vi "Read Config.vi"(8 "error in (no error)":errorcluster, 11 "Path":path) -> (0 "error out":errorcluster, 2 "Config":T1, 3 "File Created?":bool)   [LabVIEW 2020, in "MacroAssert.lvlib"]
doc: "Reads a config file located at <B>Path</B>."
uses:
  MacroAssert.lvlib
  <vilib>/Utility/config.llb/NI_LVConfig.lvlib
  <vilib>/Utility/config.llb/Read Key (String).vi
  <vilib>/Utility/config.llb/Read Key (Boolean).vi
  47c2853d-7b17-467a-9fa3-88740836eac2.vi
  CTLs/Config Key.ctl
  CTLs/Config.ctl
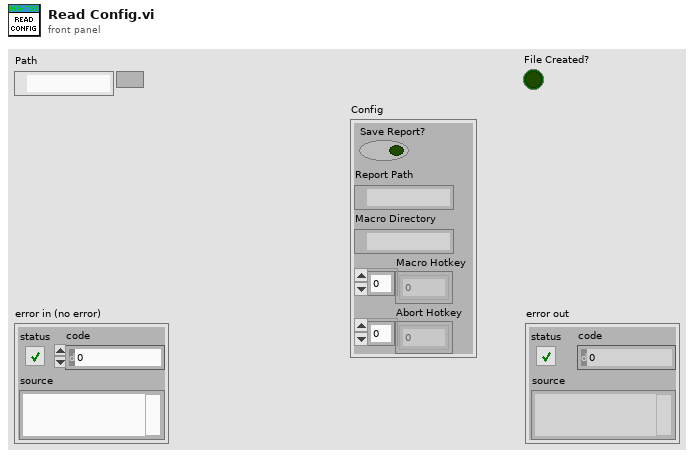
[diagram p1: front panel]
types:
  T1 = typedef "MacroAssert.lvlib/Config.ctl" = cluster{"Save Report?":bool, "Report Path":path, "Macro Directory":path, "Macro Hotkey":enum16{"0", "1", "2", "3", "4", "5", "6", "7", "8", "9", "A", "B", "C", "D", "E", "F", "G", "H", "I", "J", "K", "L", "M", "N", "O", "P", "Q", "R", "S", "T", "U", "V", "W", "X", "Y", "Z", "F1", "F2", "F3", "F4", "F5", "F6", "F7", "F8", "F9", "F10", "F11", "F12", "F13", "F14", "F15", "ADD", "BACK", "BACKSLASH", "CAPITAL", "COMMA", "DECIMAL", "DELETE", "DIVIDE", "DOWN", "END", "EQUALS", "ESCAPE", "GRAVE (`)", "HOME", "INSERT", "LBRACKET", "LCONTROL", "LEFT", "L ALT", "LSHIFT", "LWIN", "MINUS", "MULTIPLY", "NEXT", "NUMLOCK", "NUMPAD_0", "NUMPAD_1", "NUMPAD_2", "NUMPAD_3", "NUMPAD_4", "NUMPAD_5", "NUMPAD_6", "NUMPAD_7", "NUMPAD_8", "NUMPAD_9", "PAUSE", "PERIOD", "PRIOR (PG UP)", "RBRACKET", "RCONTROL", "RETURN", "RIGHT", "R ALT", "RSHIFT", "RWIN", "SCROLL", "SEMICOLON", "SLASH", "SPACE", "SUBTRACT", "TAB", "UP", "ENTER (num pad)", "' (quote)"}[], "Abort Hotkey":enum16{"0", "1", "2", "3", "4", "5", "6", "7", "8", "9", "A", "B", "C", "D", "E", "F", "G", "H", "I", "J", "K", "L", "M", "N", "O", "P", "Q", "R", "S", "T", "U", "V", "W", "X", "Y", "Z", "F1", "F2", "F3", "F4", "F5", "F6", "F7", "F8", "F9", "F10", "F11", "F12", "F13", "F14", "F15", "ADD", "BACK", "BACKSLASH", "CAPITAL", "COMMA", "DECIMAL", "DELETE", "DIVIDE", "DOWN", "END", "EQUALS", "ESCAPE", "GRAVE (`)", "HOME", "INSERT", "LBRACKET", "LCONTROL", "LEFT", "L ALT", "LSHIFT", "LWIN", "MINUS", "MULTIPLY", "NEXT", "NUMLOCK", "NUMPAD_0", "NUMPAD_1", "NUMPAD_2", "NUMPAD_3", "NUMPAD_4", "NUMPAD_5", "NUMPAD_6", "NUMPAD_7", "NUMPAD_8", "NUMPAD_9", "PAUSE", "PERIOD", "PRIOR (PG UP)", "RBRACKET", "RCONTROL", "RETURN", "RIGHT", "R ALT", "RSHIFT", "RWIN", "SCROLL", "SEMICOLON", "SLASH", "SPACE", "SUBTRACT", "TAB", "UP", "ENTER (num pad)", "' (quote)"}[]}
  T2 = typedef "MacroAssert.lvlib/Config Key.ctl" = enum16{"SaveReport", "ReportPath", "MacroDirectory", "MacroHotkey", "AbortHotkey"}
  T3 = typedef "NI_LVConfig.lvlib/Config Data RefNum.ctl" = refnum<k1>
  T4 = enum16{"0", "1", "2", "3", "4", "5", "6", "7", "8", "9", "A", "B", "C", "D", "E", "F", "G", "H", "I", "J", "K", "L", "M", "N", "O", "P", "Q", "R", "S", "T", "U", "V", "W", "X", "Y", "Z", "F1", "F2", "F3", "F4", "F5", "F6", "F7", "F8", "F9", "F10", "F11", "F12", "F13", "F14", "F15", "ADD", "BACK", "BACKSLASH", "CAPITAL", "COMMA", "DECIMAL", "DELETE", "DIVIDE", "DOWN", "END", "EQUALS", "ESCAPE", "GRAVE (`)", "HOME", "INSERT", "LBRACKET", "LCONTROL", "LEFT", "L ALT", "LSHIFT", "LWIN", "MINUS", "MULTIPLY", "NEXT", "NUMLOCK", "NUMPAD_0", "NUMPAD_1", "NUMPAD_2", "NUMPAD_3", "NUMPAD_4", "NUMPAD_5", "NUMPAD_6", "NUMPAD_7", "NUMPAD_8", "NUMPAD_9", "PAUSE", "PERIOD", "PRIOR (PG UP)", "RBRACKET", "RCONTROL", "RETURN", "RIGHT", "R ALT", "RSHIFT", "RWIN", "SCROLL", "SEMICOLON", "SLASH", "SPACE", "SUBTRACT", "TAB", "UP", "ENTER (num pad)", "' (quote)"}[]
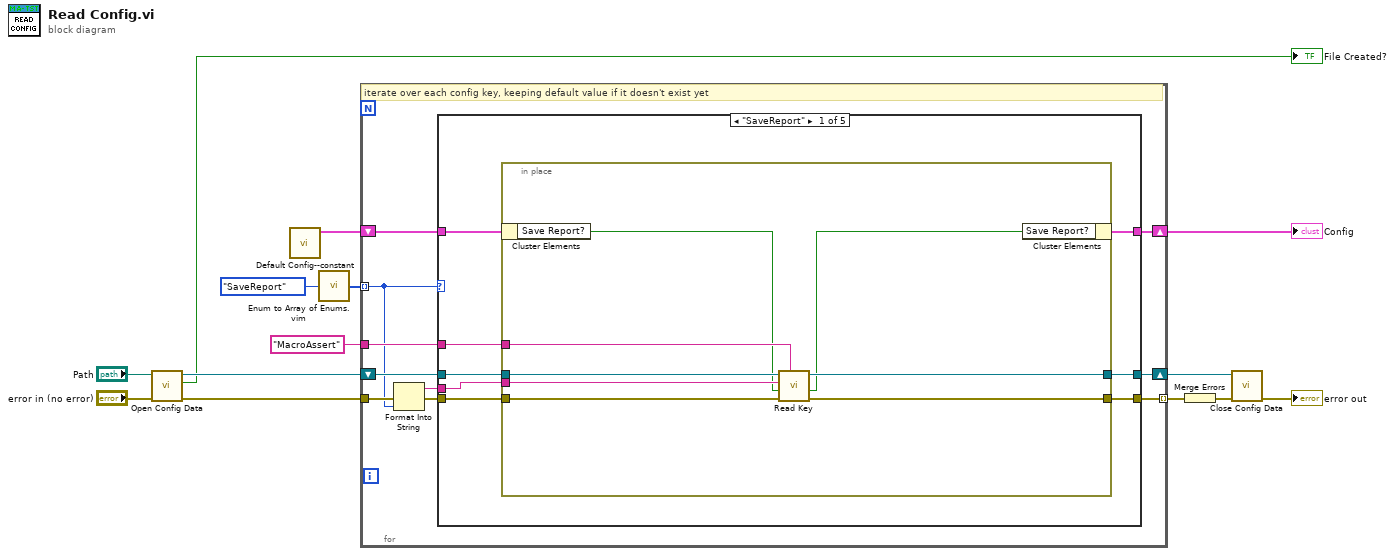
[diagram p0: block diagram]
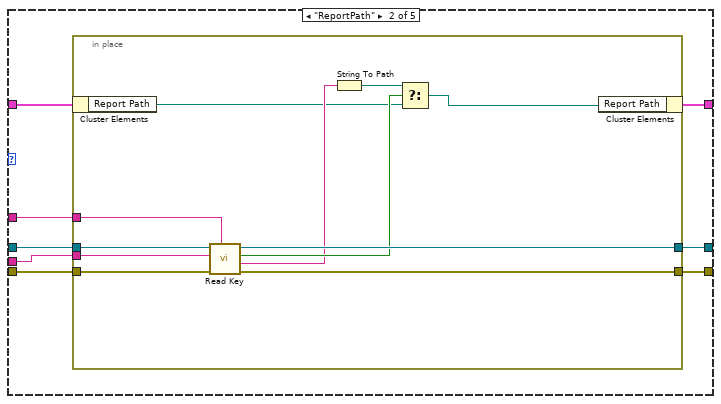
[diagram p2: hidden frame]
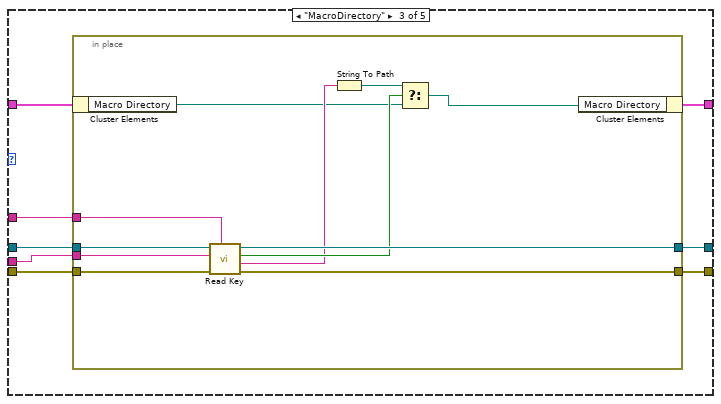
[diagram p3: hidden frame]
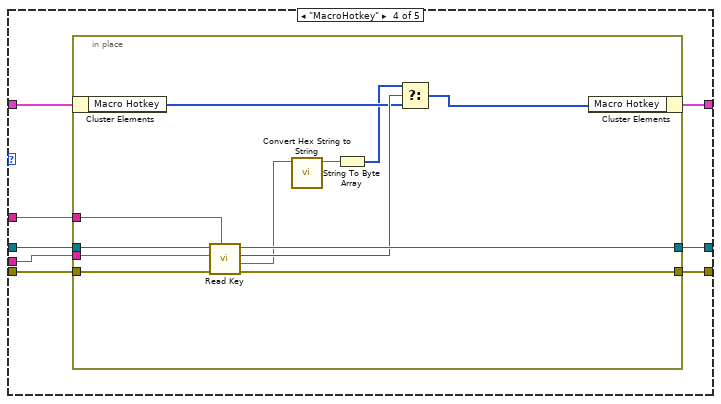
[diagram p4: hidden frame]
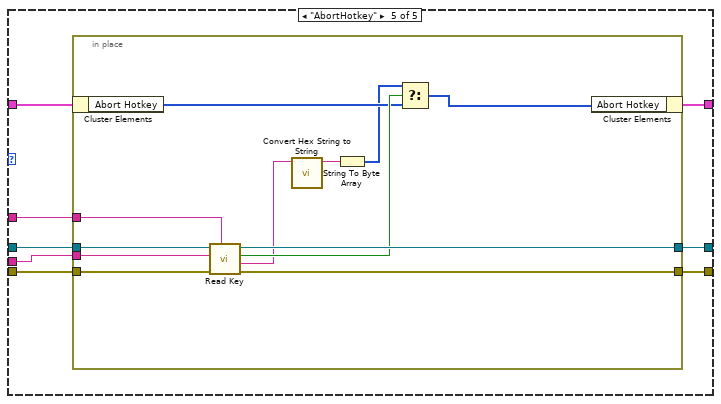
[diagram p5: hidden frame]
diagram:
  n1 = call <vilib>:"Open Config Data.vi"("error in (no error)"="error in (no error)", "configuration file path"="Path") -> ("error out"=w11:errorcluster, "file created?"=→"File Created?":bool, "refnum"=w14:T3)  [unwired: 7 in]
  n2 = call "Default Config--constant.vi"() -> ("Default Config"=w2:T1)  [unwired: 11 in]
  n3 = call "Enum to Array of Enums.vim"("enum"=Config_Key."SaveReport" ("Config Key")) -> ("array of enums"=w7:T2[])
  n4 = for {
    tunnel: w7 -> [w15] mode=indexing
    shift-right: [w18] -> w1
    shift-left: w2 -> [w21]
    tunnel: "MacroAssert" ("section") -> [w20]
    tunnel: [w23] -> w5 mode=indexing
    tunnel: w11 -> [w22]
    shift-right: [w16] -> w4
    shift-left: w14 -> [w17]
    # "iterate over each config key, keeping default value if it doesn't exist yet"
    n5 = Format Into String(error in=w22, w15) -> (resulting string=w19:string, error out=w24:errorcluster)  [unwired: 2 in]
    n6 = case shown="\"SaveReport\"" w15 {
      tunnel: w21 -> [w28 w44 w63 w82 w102]
      tunnel: w20 -> [w29 w45 w64 w83 w103]
      tunnel: w19 -> [w30 w46 w65 w84 w104]
      tunnel: w24 -> [w32 w48 w67 w86 w106]
      tunnel: [w31 w47 w66 w85 w105] -> w23
      tunnel: [w27 w43 w62 w81 w101] -> w18
      tunnel: w17 -> [w26 w42 w61 w80 w100]
      tunnel: [w25 w41 w60 w79 w99] -> w16
      frame "SaveReport" {
        n7 = in-place {
          in-place-border: w30 -> [w37]
          in-place-border: w32 -> [w40]
          in-place-border: w29 -> [w36]
          in-place-border: [w39] -> w31
          in-place-border: w26 -> [w35]
          in-place-border: [w38] -> w25
          n8 = in-place-cluster #1(w28) -> ("Save Report?"=w34:bool)
          n9 = call-poly <vilib>:"Read Key.vi"("section"=w36, "error in (no error)"=w40, "default value"=w34, "key"=w37, "refnum"=w35) -> ("error out"=w39:errorcluster, "value"=w33:bool, "refnum out"=w38:T3)  [unwired: 3 in, 1 out]
          n10 = in-place-cluster #1("Save Report?"=w33) -> (w27:T1)
        }
      }
      frame "ReportPath" {
        n11 = in-place {
          in-place-border: w46 -> [w56]
          in-place-border: w48 -> [w59]
          in-place-border: w45 -> [w55]
          in-place-border: [w58] -> w47
          in-place-border: w42 -> [w49]
          in-place-border: [w57] -> w41
          n12 = in-place-cluster #2(w44) -> ("Report Path"=w51:path)
          n13 = call-poly <vilib>:"Read Key.vi"("section"=w55, "error in (no error)"=w59, "key"=w56, "refnum"=w49) -> ("error out"=w58:errorcluster, "value"=w52:string, "found?"=w54:bool, "refnum out"=w57:T3)  [unwired: 4 in]
          n14 = String To Path(string=w52) -> (path=w53:path)
          n15 = Select(t=w53, s=w54, f=w51) -> (s? t:f=w50:path)
          n16 = in-place-cluster #2("Report Path"=w50) -> (w43:T1)
        }
      }
      frame "MacroDirectory" {
        n17 = in-place {
          in-place-border: w65 -> [w75]
          in-place-border: w67 -> [w78]
          in-place-border: w64 -> [w74]
          in-place-border: [w77] -> w66
          in-place-border: w61 -> [w68]
          in-place-border: [w76] -> w60
          n18 = in-place-cluster #3(w63) -> ("Macro Directory"=w70:path)
          n19 = call-poly <vilib>:"Read Key.vi"("section"=w74, "error in (no error)"=w78, "key"=w75, "refnum"=w68) -> ("error out"=w77:errorcluster, "value"=w71:string, "found?"=w73:bool, "refnum out"=w76:T3)  [unwired: 4 in]
          n20 = String To Path(string=w71) -> (path=w72:path)
          n21 = Select(t=w72, s=w73, f=w70) -> (s? t:f=w69:path)
          n22 = in-place-cluster #3("Macro Directory"=w69) -> (w62:T1)
        }
      }
      frame "MacroHotkey" {
        n23 = in-place {
          in-place-border: w84 -> [w95]
          in-place-border: w86 -> [w98]
          in-place-border: w83 -> [w94]
          in-place-border: [w97] -> w85
          in-place-border: w80 -> [w90]
          in-place-border: [w96] -> w79
          n24 = in-place-cluster #4(w82) -> ("Macro Hotkey"=w92:T4)
          n25 = call-poly <vilib>:"Read Key.vi"("section"=w94, "error in (no error)"=w98, "key"=w95, "refnum"=w90) -> ("error out"=w97:errorcluster, "value"=w89:string, "found?"=w93:bool, "refnum out"=w96:T3)  [unwired: 4 in]
          n26 = call "Convert Hex String to String.vi"("Hex String"=w89) -> ("String"=w88:string)  [unwired: 10 in]
          n27 = String To Byte Array(string=w88) -> (unsigned byte array=w87:u8[])
          n28 = Select(t=w87, s=w93, f=w92) -> (s? t:f=w91:u16[])
          n29 = in-place-cluster #4("Macro Hotkey"=w91) -> (w81:T1)
        }
      }
      frame "AbortHotkey" {
        n30 = in-place {
          in-place-border: w104 -> [w115]
          in-place-border: w106 -> [w118]
          in-place-border: w103 -> [w114]
          in-place-border: [w117] -> w105
          in-place-border: w100 -> [w110]
          in-place-border: [w116] -> w99
          n31 = in-place-cluster #5(w102) -> ("Abort Hotkey"=w112:T4)
          n32 = call-poly <vilib>:"Read Key.vi"("section"=w114, "error in (no error)"=w118, "key"=w115, "refnum"=w110) -> ("error out"=w117:errorcluster, "value"=w109:string, "found?"=w113:bool, "refnum out"=w116:T3)  [unwired: 4 in]
          n33 = call "Convert Hex String to String.vi"("Hex String"=w109) -> ("String"=w108:string)  [unwired: 10 in]
          n34 = String To Byte Array(string=w108) -> (unsigned byte array=w107:u8[])
          n35 = Select(t=w107, s=w113, f=w112) -> (s? t:f=w111:u16[])
          n36 = in-place-cluster #5("Abort Hotkey"=w111) -> (w101:T1)
        }
      }
    }
  }
  "Config" <- w1
  n37 = Merge Errors(w5) -> (w10:errorcluster)
  n38 = call <vilib>:"Close Config Data.vi"("error in (no error)"=w10, "refnum"=w4) -> ("error out"=→"error out":errorcluster)  [unwired: 8 in, 1 out]
